vi "Pre-Build Action.vi"(6 "Top Level/Always Included VIs":path[](array[path]), 7 "Main Destination Path":path, 9 "Target Name":string, 10 "Build Specification Name":string, 11 "Project Path":path) -> (0 "error out":errorcluster)   [LabVIEW 2020]
uses:
  3b58ec78-2b4e-4f6e-811a-c079fee85fd5.vi
  <vilib>/Comparison/Equal/Equal Functor/Equal Functor.lvclass
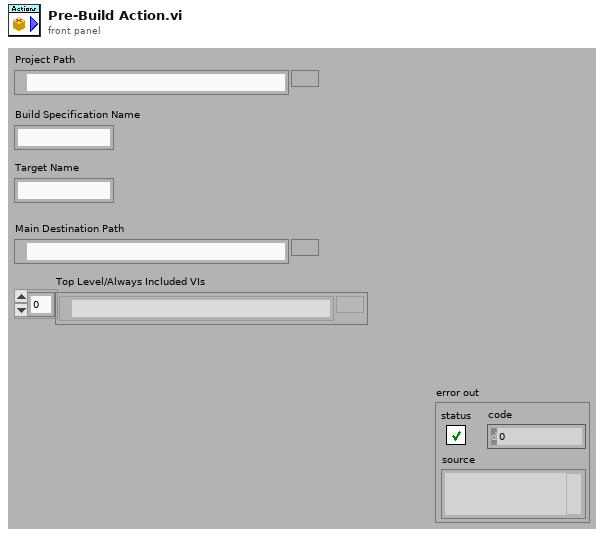
[diagram p1: front panel]
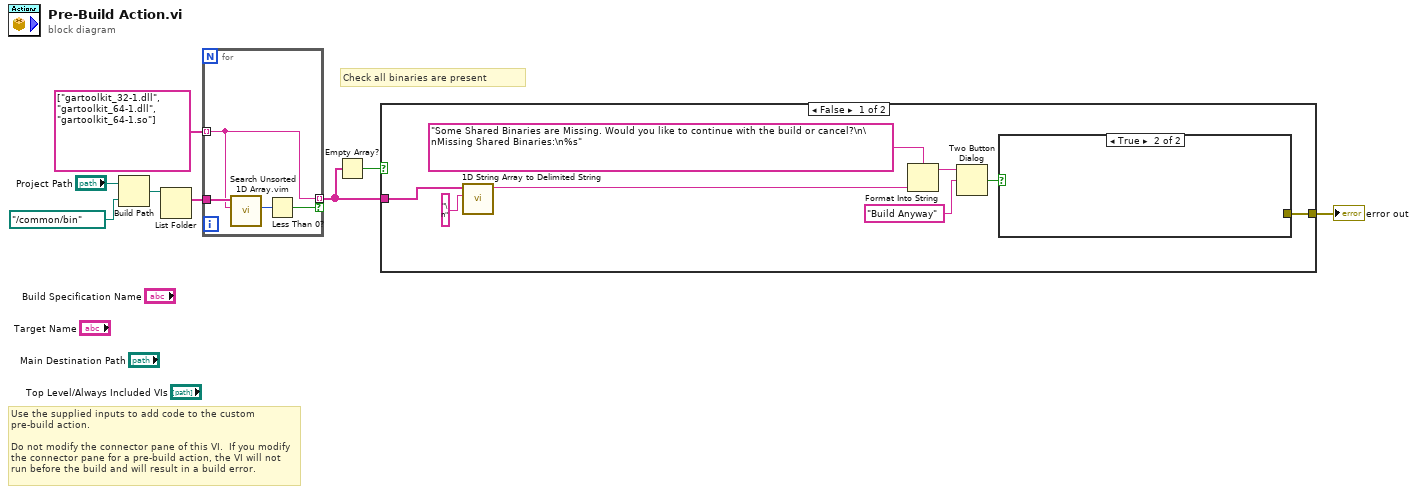
[diagram p0: block diagram]
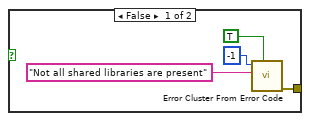
[diagram p2: hidden frame]
diagram:
  # "Check all binaries are present"
  # "Use the supplied inputs to add code to the custom pre-build action.\n\nDo not modify the connector pane of this VI.  If you modify the connector pane for a pre-build action, the VI will not run before the build and will result in a build error."
  n1 = Build Path(base path="Project Path", name or relative path=path "../common/bin") -> (appended path=w6:path)
  n2 = List Folder(path=w6) -> (filenames=w5:string[])  [unwired: 3 in, 3 out]
  n3 = for {
    tunnel: w5 -> [w12]
    tunnel: string[] ["gartoolkit_32-1.dll", "gartoolkit_64-1.dll", "gartoolkit_64-1.so"] ("Path") -> [w10] mode=indexing
    tunnel: [w10] -> w1 mode=indexing if=w9
    n4 = call "Search Unsorted 1D Array.vim"("element"=w10, "unsorted 1D array"=w12) -> ("index of element"=w11:i32)  [unwired: 9 in]
    n5 = Less Than 0?(x=w11) -> (x < 0?=w9:bool)
  }
  n6 = Empty Array?(array=w1) -> (empty?=w3:bool)
  n7 = case shown="False" w3 {
    tunnel: [w20 _] -> w2
    tunnel: w1 -> [w19 _]
    frame False {
      n8 = call <vilib>:"1D String Array to Delimited String.vi"("delimiter"="\n", "string array"=w19) -> ("delimited string"=w17:string)  [unwired: 9 in]
      n9 = Format Into String(format string="Some Shared Binaries are Missing. Would you like to continue with the build or cancel?\n\nMissing Shared Binaries:\n%s", w17) -> (resulting string=w16:string)  [unwired: 2 in, 1 out]
      n10 = Two Button Dialog(message=w16, 2:"Build Anyway" ("T button name (\"OK\")")) -> (T button?=w14:bool)  [unwired: 1 in]
      n11 = case shown="True" w14 {
        tunnel: [w24 _] -> w20
        frame False {
          n12 = call <vilib>:"Error Cluster From Error Code.vi"("show call chain? (False)"=TRUE, "error message (\"\")"="Not all shared libraries are present" ("error message (\"\")"), "error code (0)"=-1) -> ("error out"=w24:errorcluster)  [unwired: 6 in]
        }
        frame True {
        }
      }
    }
    frame True {
    }
  }
  "error out" <- w2
